vi "Build_ACQ_cfg.vi"(1 "User Event in":refnum<user-event>, 2 "Audio Settings":T4, 3 "Audio Device Details":T1(array[cluster])) -> (0 "Audio DAQ cfg":T2)   [LabVIEW 2020]
uses:
  typedefs/Audio_Data.ctl
  <vilib>/sound2/lvsound2.llb/Sound Data Format.ctl
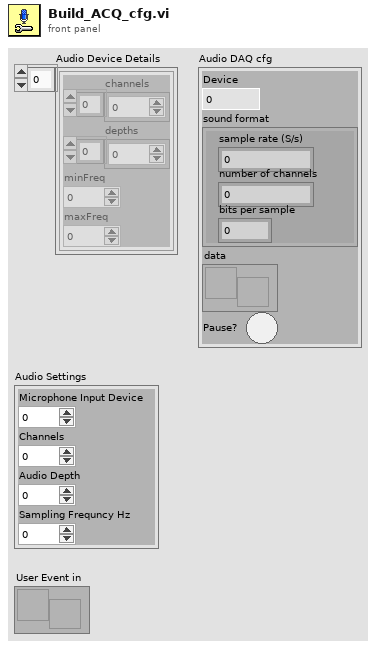
[diagram p1: front panel]
types:
  T1 = cluster{"channels":i32[], "depths":i32[], "minFreq":dbl, "maxFreq":dbl}[]
  T2 = typedef "Audio_Data.ctl" = cluster{"Device":u32, "sound format":T3, "data":refnum<user-event>, "Pause?":bool}
  T3 = typedef "Sound Data Format.ctl" = cluster{"sample rate (S/s)":dbl, "number of channels":i32, "bits per sample":i32}
  T4 = cluster{"Microphone Input Device":u32, "Channels":i32, "Audio Depth":i32, "Sampling Frequncy Hz":dbl}
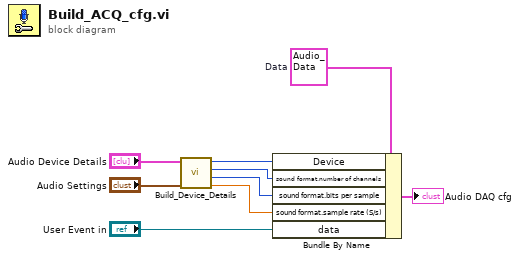
[diagram p0: block diagram]
diagram:
  w7 = T2 {"Device"=0, "sound format"={"sample rate (S/s)"=22050.0, "number of channels"=2, "bits per sample"=16}, "data"=refnum, "Pause?"=FALSE}  # Data
  n1 = call "Build_Device_Details.vi"("Audio Settings"="Audio Settings", "Audio Device Details"="Audio Device Details") -> ("Sampling Frequncy Hz"=w1:dbl, "Depth"=w2:i32, "Channel"=w3:i32, "Device ID"=w4:u32)  [unwired: 4 in, 2 out]
  n2 = Bundle By Name(cluster=w7, "Device"=w4, "sound format.number of channels"=w3, "sound format.bits per sample"=w2, "sound format.sample rate (S/s)"=w1, "data"="User Event in") -> (→"Audio DAQ cfg":T2)
